vi "Mag_Read .vi"(0 "I2CDevRef":T1 {"Device Address" format="%.0x"}, 5 "Sensitivity X/Y":i32(ring) items=["+/- 1.3"=1100, "+/-1.9"=855, "+/-2.5"=670, "+/-4.0"=450, "+/-4.7"=400, "+/-5.6"=330, "+/-8.1"=230], 7 "Sensitivity Z":i32(ring) items=["+/- 1.3"=980, "+/-1.9"=760, "+/-2.5"=600, "+/-4.0"=400, "+/-4.7"=355, "+/-5.6"=296, "+/-8.1"=205], 9 "Axis":string, 11 "error in":errorcluster) -> (4 "I2CDevRef Out":T1 {"Device Address" format="%.0x"}, 6 "Heading":i32, 8 "x+y":i16, 15 "error out":errorcluster)   [LabVIEW 2011]
uses:
  <vilib>/Rock Robotics/WPI/I2C/WPI_I2CDevRef.ctl
  <vilib>/Rock Robotics/SystemInterfaces/Typedef/FPGA_TypedefDigitalModule.ctl
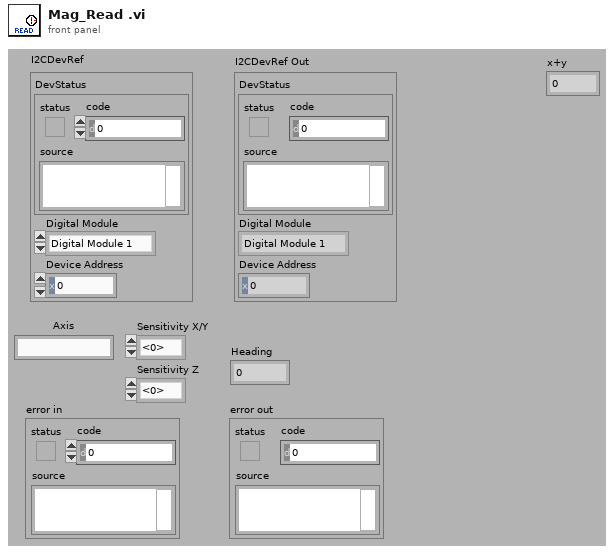
[diagram p1: front panel]
types:
  T1 = typedef "WPI_I2CDevRef.ctl" = cluster{"DevStatus":errorcluster, "Digital Module":T2, "Device Address":u8}
  T2 = typedef "FPGA_TypedefDigitalModule.ctl" = enum16{"Digital Module 1", "Digital Module 2"}
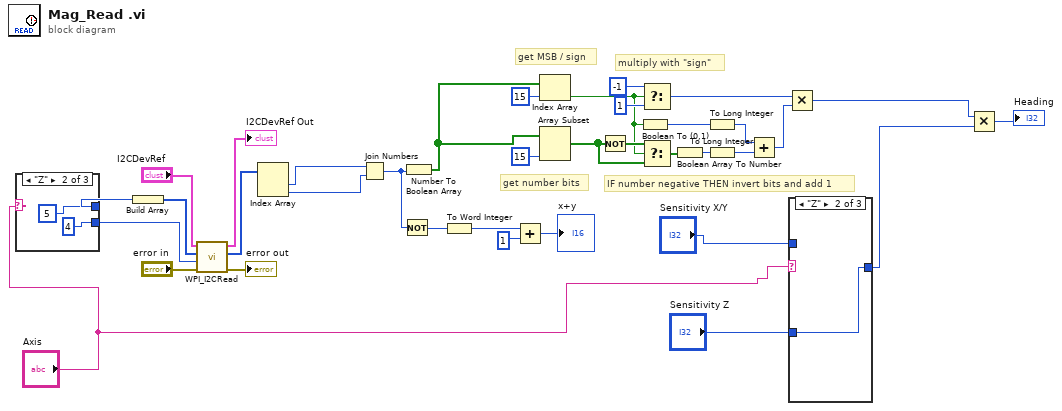
[diagram p0: block diagram]
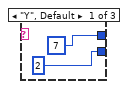
[diagram p4: hidden frame]
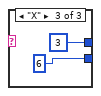
[diagram p5: hidden frame]
diagram:
  # "multiply with \"sign\""
  # "IF number negative THEN invert bits and add 1"
  # "get number bits"
  # "get MSB / sign"
  n1 = case shown="\"Z\"" "Axis" {
    tunnel: [u8 7 ("Data To Send") u8 5 ("Data To Send") u8 3 ("Data To Send")] -> w30
    tunnel: [u8 2 ("I2CBytesToRead") u8 4 ("I2CBytesToRead") u8 6 ("I2CBytesToRead")] -> w1
    frame "Y", Default {
    }
    frame "Z" {
    }
    frame "X" {
    }
  }
  n2 = Build Array(w30) -> (w32:u8[])
  n3 = call <vilib>:"WPI_I2CRead.vi"("error in (no error)"="error in", "I2CBytesToRead"=w1, "I2CRegister"=w32, "I2CDevRef"="I2CDevRef") -> ("error out"=→"error out":errorcluster, "Data Out"=w33:u8[], "I2CDevRef"=→"I2CDevRef Out":T1)  [unwired: 1 in, 4 out]
  n4 = Index Array(array=w33) -> (element #1=w28:u8, element #2=w27:u8)  [unwired: 2 in]
  n5 = Join Numbers(hi=w28, lo=w27) -> ((hi.lo)=w3:u16)
  n6 = Not(x=w3) -> (.not. x?=w4:u16)
  n7 = Number To Boolean Array(number=w3) -> (Boolean array=w12:bool[])
  n8 = To Word Integer(number=w4) -> (16bit integer=w5:i16)
  n9 = Add(x=w5, y=i16 1) -> (x+y=→"x+y":i16)
  n10 = Index Array(array=w12, index=15) -> (element=w15:bool)
  n11 = Array Subset(array=w12, length=15) -> (w14:bool[])  [unwired: 1 in]
  n12 = Not(x=w14) -> (.not. x?=w23:bool[])
  n13 = Boolean To (0,1)(Boolean=w15) -> (0, 1=w21:i16)
  n14 = Select(t=-1, s=w15, f=1) -> (s? t:f=w18:i32)
  n15 = Select(t=w23, s=w15, f=w14) -> (s? t:f=w13:bool[])
  n16 = Boolean Array To Number(Boolean array=w13) -> (number=w24:u32)
  n17 = To Long Integer(number=w21) -> (32bit integer=w16:i32)
  n18 = To Long Integer(number=w24) -> (32bit integer=w22:i32)
  n19 = Add(x=w16, y=w22) -> (x+y=w17:i32)
  n20 = Multiply(x=w18, y=w17) -> (x*y=w11:i32)
  n21 = case shown="\"Z\"" "Axis" {
    tunnel: [w43 w44 w45] -> w7
    tunnel: "Sensitivity X/Y" -> [w43 _ w45]
    tunnel: "Sensitivity Z" -> [_ w44 _]
    frame "Y", Default {
    }
    frame "Z" {
    }
    frame "X" {
    }
  }
  n22 = Multiply(x=w11, y=w7) -> (x*y=→"Heading":i32)
